vi "test_csvBitShift.vi"() -> ()   [LabVIEW 2017]
uses:
  <vilib>/Utility/file.llb/Read Delimited Spreadsheet (DBL).vi
panel:
  out "integer":i16
  out "interleaved array":fxp<+/-,16,5>[](array[numeric])
  in  "reference traj path":path=path "C:/Users/arnold/Documents/labview/afm_imaging/data/data-in.csv"
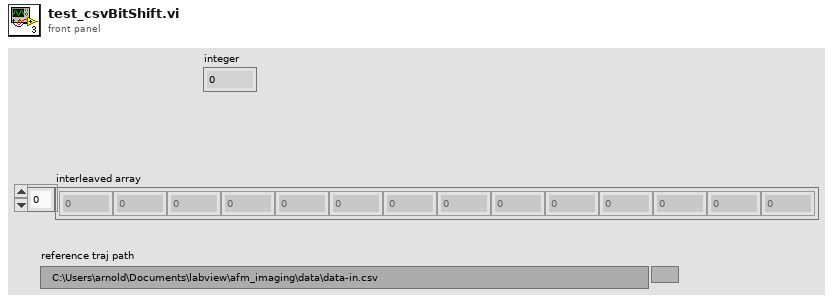
[diagram p1: front panel]
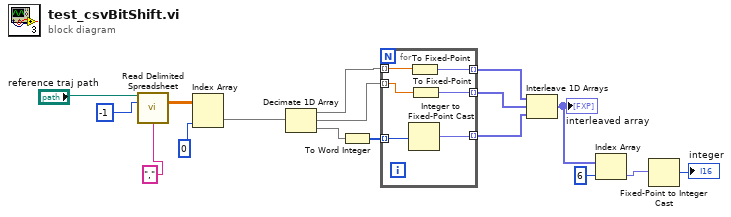
[diagram p0: block diagram]
diagram:
  n1 = call-poly <vilib>:"Read Delimited Spreadsheet.vi"("file path (dialog if empty)"="reference traj path", "number of rows (all:-1)"=-1, "delimiter (\\t)"=",") -> ("all rows"=w13:dbl[][])  [unwired: 7 in, 5 out]
  n2 = Index Array(array=w13, index (col)=0 ("dimension size")) -> (element=w12:dbl[])  [unwired: 1 in]
  n3 = Decimate 1D Array(w12) -> (w10:dbl[], w9:dbl[], w11:dbl[])
  n4 = To Word Integer(number=w11) -> (16bit integer=w8:i16[])
  n5 = for {
    tunnel: w10 -> [w23] mode=indexing
    tunnel: w9 -> [w22] mode=indexing
    tunnel: [w21] -> w6 mode=indexing
    tunnel: [w20] -> w7 mode=indexing
    tunnel: w8 -> [w19] mode=indexing
    tunnel: [w18] -> w5 mode=indexing
    n6 = Integer to Fixed-Point Cast(integer=w19) -> (fixed-point=w18:fxp<+/-,16,5>)  [unwired: 1 in]
    n7 = To Fixed-Point(number=w23) -> (fixed-point=w20:fxp<+/-,16,5>)  [unwired: 1 in]
    n8 = To Fixed-Point(number=w22) -> (fixed-point=w21:fxp<+/-,16,5>)  [unwired: 1 in]
  }
  n9 = Interleave 1D Arrays(w7, w6, w5) -> (w4:fxp<+/-,16,5>[])
  "interleaved array" <- w4
  n10 = Index Array(array=w4, index=6) -> (element=w3:fxp<+/-,16,5>)
  n11 = Fixed-Point to Integer Cast(1:w3) -> (0:→"integer":i16)
